vi "Init.vi"(8 "error in (no error)":errorcluster, 11 "Report Generator In":refnum<class "Result Collector.lvclass">) -> (0 "error out":errorcluster, 3 "Report Generator Out":refnum<class "Result Collector.lvclass">)   [LabVIEW 2020, in "Result Collector.lvclass"]
uses:
  Result Collector.lvclass
  Result Types/Assertion Result/Public/TypeDefs/Status.ctl
  Result Types/Assertion Result/Assertion Result.lvlib
  Result Types/Assertion Result/Public/TypeDefs/Assertion Type.ctl
  Result Types/Assertion Result/Assertion Result.ctl
  Result Types/Method Result/Method Result.ctl
  Result Types/Method Result/Method Result.lvlib
  Result Types/Case Result/Test Case Result.ctl
  Result Types/Case Result/Test Case Result.lvlib
  Result Types/Suite Results/Test Suite Result.ctl
  Result Types/Suite Results/Test Suite Result.lvlib
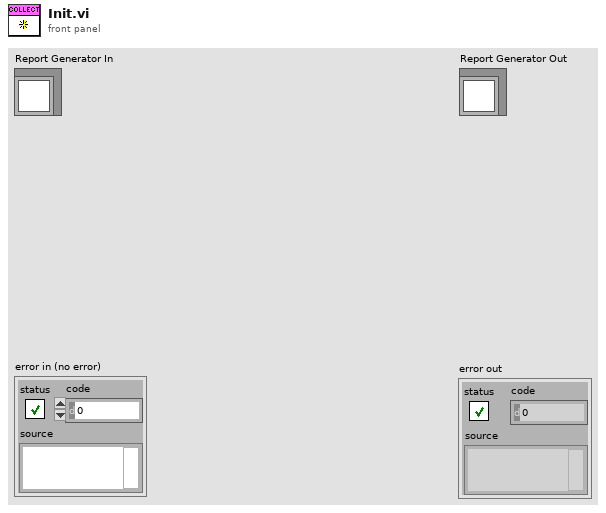
[diagram p1: front panel]
types:
  T1 = typedef "Test Case Result.lvlib/Test Case Result.ctl" = map{string, T2}
  T2 = typedef "Method Result.lvlib/Method Result.ctl" = cluster{"Test Case":string, "Test Method Name":string, "Status":T3, "Assertion Results":T4[], "Execution time":dbl, "Result String":string}
  T3 = typedef "Assertion Result.lvlib/Status.ctl" = enum16{"Pass", "Fail", "Error", "Skipped", "Setup Error", "Broken", "Teardown Error"}
  T4 = typedef "Assertion Result.lvlib/Assertion Result.ctl" = cluster{"Status":T3, "Message":string, "Description":string, "Assertion Type":T5}
  T5 = typedef "Assertion Result.lvlib/Assertion Type.ctl" = enum16{"None", "Pass", "Fail", "Skip", "Pass if Equal", "Fail if Equal", "Pass if Error", "Fail if Error", "Pass if", "Fail if"}
  T6 = typedef "Test Suite Result.lvlib/Test Suite Result.ctl" = cluster{"Test Suite ID":string, "Name":string, "Hostname":string, "Status":T3, "Execution time":dbl, "Start Time":timestamp, "Case Results":T1[]}
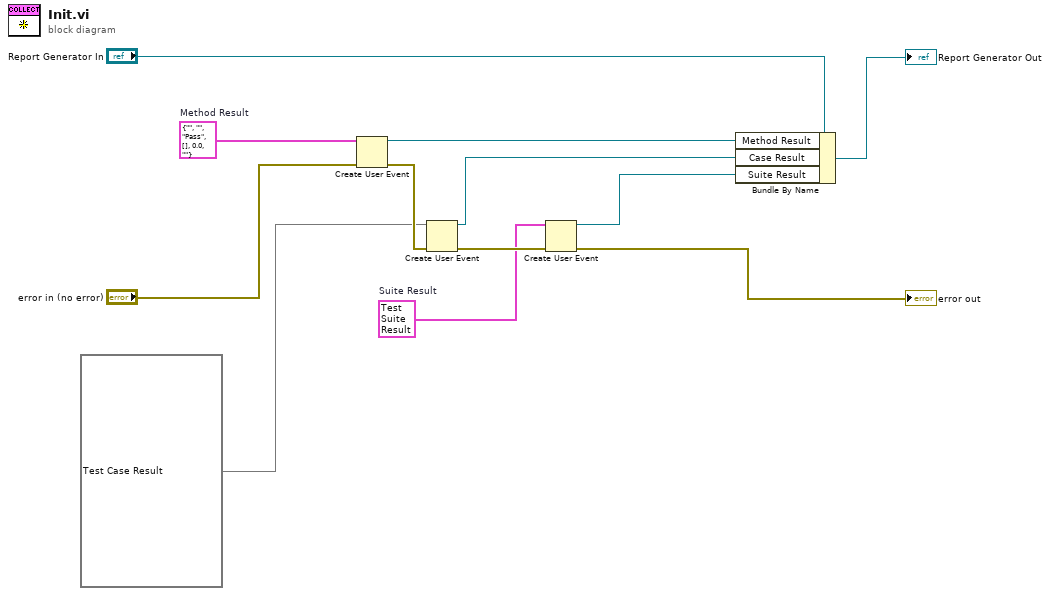
[diagram p0: block diagram]
diagram:
  w6 = T2 {"Test Case"="", "Test Method Name"="", "Status"=enum."Pass", "Assertion Results"=[], "Execution time"=0.0, "Result String"=""}  # Method Result
  w8 = T6 {"Test Suite ID"="", "Name"="", "Hostname"="", "Status"=enum."Pass", "Execution time"=0.0, "Start Time"=timestamp(0 s since 1904-01-01), "Case Results"=[]}  # Suite Result
  n1 = Create User Event(user event datatype=w6, error in="error in (no error)") -> (user event=w4:refnum<user-event>, error out=w10:errorcluster)
  n2 = Create User Event(user event datatype=T1 {} ("Method Results"), error in=w10) -> (user event=w3:refnum<user-event>, error out=w9:errorcluster)
  n3 = Create User Event(user event datatype=w8, error in=w9) -> (user event=w2:refnum<user-event>, error out=→"error out":errorcluster)
  n4 = Bundle By Name(cluster="Report Generator In", "Method Result"=w4, "Case Result"=w3, "Suite Result"=w2) -> (→"Report Generator Out":refnum<class "Result Collector.lvclass">)
